vi "start.vi"() -> ()   [LabVIEW 2016]
panel:
  out "Array":errorcluster[](array[cluster])
  in  "error in (no error) 2":errorcluster
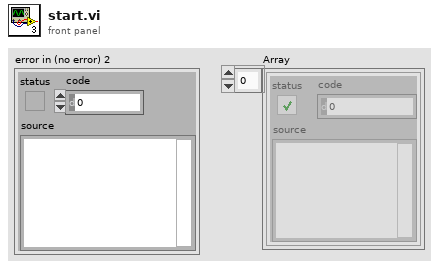
[diagram p1: front panel]
types:
  T1 = typedef "LVAllMonitorsDisplayTypeDef.ctl" = cluster{"Bounds":cluster{"Left":i16, "Top":i16, "Right":i16, "Bottom":i16}, "Depth":i16}[]
  T2 = cluster{"Left":i16, "Top":i16, "Right":i16, "Bottom":i16}
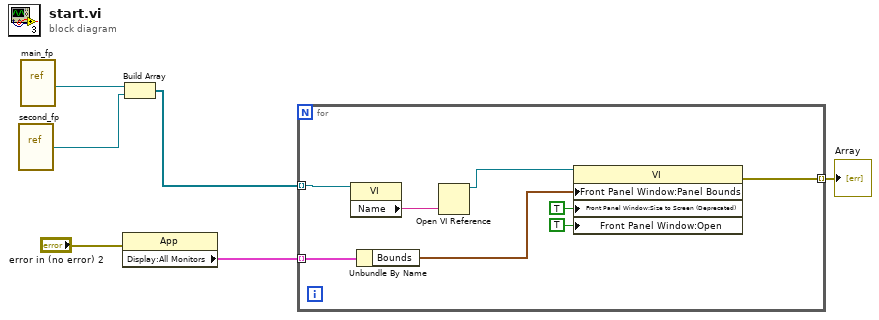
[diagram p0: block diagram]
diagram:
  n1 = vi-ref "second_fp.vi"() -> (w5:refnum<vi>)
  n2 = vi-ref "main_fp.vi"() -> (w6:refnum<vi>)
  n3 = property class="App"(error in="error in (no error) 2") -> ("Display:All Monitors"=w3:T1)  [unwired: 1 in, 2 out]
  n4 = Build Array(w6, w5) -> (w2:refnum<vi>[])
  n5 = for {
    tunnel: w3 -> [w12] mode=indexing
    tunnel: w2 -> [w13] mode=indexing
    tunnel: [w7] -> w1 mode=indexing
    n6 = property class="VI"(reference=w13) -> ("Name"=w14:string)  [unwired: 1 in, 2 out]
    n7 = Unbundle By Name(w12) -> ("Bounds"=w10:T2)
    n8 = Open VI Reference(vi path=w14) -> (vi reference=w11:refnum<vi>)  [unwired: 5 in, 1 out]
    n9 = property class="VI"(reference=w11, "Front Panel Window:Panel Bounds"=w10, "Front Panel Window:Size to Screen (Deprecated)"=TRUE, "Front Panel Window:Open"=TRUE) -> (error out=w7:errorcluster)  [unwired: 1 in, 1 out]
  }
  "Array" <- w1
